vi "Verify Borders Row.vi"(7 "Column Number":i32, 8 "error in (no error)":errorcluster, 9 "No border?":bool, 10 "Column Borders IN [ ]":T1) -> (2 "Column Borders OUT [ ]":T1)   [LabVIEW 2019, in "Exaprom PDF.lvlib" / "Pdfp Table Class.lvclass"]
doc: "Version 1.0\nDeveloped by Jean-Marc Simard\nCopyright © 2010, Exaprom Inc.\nAll rights reserved.\nLicense: BSD"
uses:
  Pdfp Table Class.lvclass
  Controls/Table Controls/Border and BG Color [ ].ctl
  Controls/Table Controls/Border and BG Color.ctl
  Controls/Table Controls/Cell Border 20 px.ctl
  Exaprom PDF.lvlib
panel:
  out "error out":errorcluster
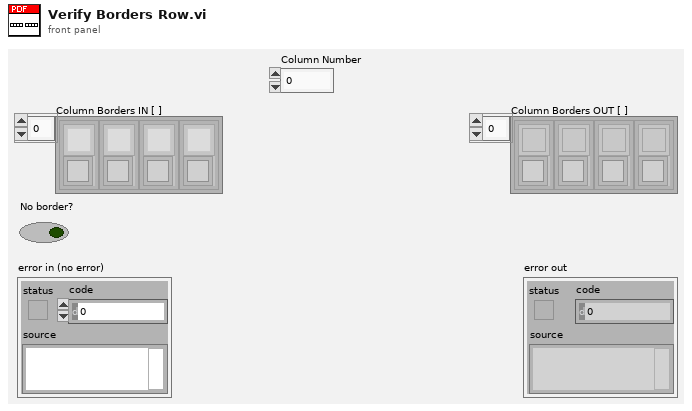
[diagram p1: front panel]
types:
  T1 = typedef "Exaprom PDF.lvlib/Border and BG Color [ ].ctl" = T2[]
  T2 = typedef "Exaprom PDF.lvlib/Border and BG Color.ctl" = cluster{"Cell Border":T3, "BG":u32}
  T3 = typedef "Exaprom PDF.lvlib/Cell Border 20 px.ctl" = u16
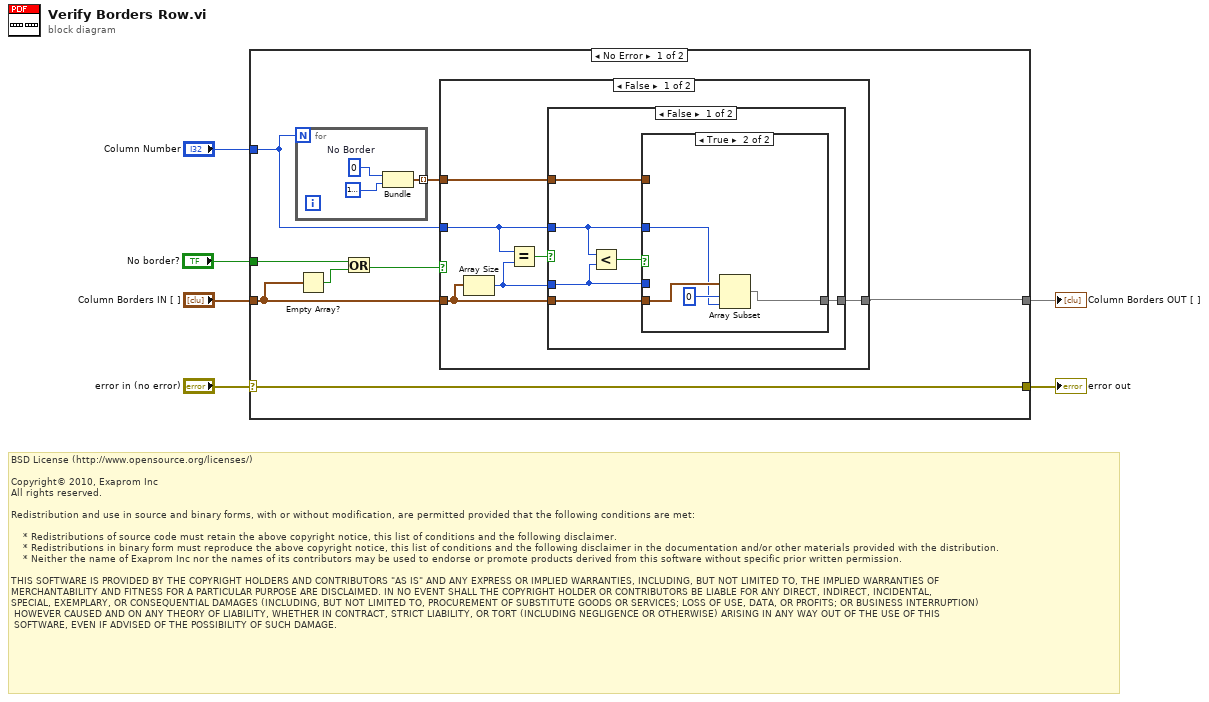
[diagram p0: block diagram]
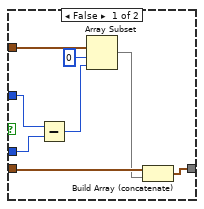
[diagram p2: hidden frame]
diagram:
  # "BSD License (http://www.opensource.org/licenses/)\n\nCopyright© 2010, Exaprom Inc\nAll rights reserved.\n\nRedistribution and use in source and binary forms, with or without modification, are permitted provided that the following conditions are met:\n\n    * Redistributions of source code must retain the above copyright notice, this list of conditions and the following disclaimer.\n    * Redistributions in binary form must reproduce the above copyright notice, this list of conditions and the following disclaimer in the documentation and/or other materials provided with the distribution.\n    * Neither the name of Exaprom Inc nor the names of its contributors may be used to endorse or promote products derived from this software without specific prior written permission.\n\nTHIS SOFTWARE IS PROVIDED BY THE COPYRIGHT HOLDERS AND CONTRIBUTORS \"AS IS\" AND ANY EXPRESS OR IMPLIED WARRANTIES, INCLUDING, BUT NOT LIMITED TO, THE IMPLIED WARRANTIES OF \nMERCHANTABILITY AND FITNESS FOR A PARTICULAR PURPOSE ARE DISCLAIMED. IN NO EVENT SHALL THE COPYRIGHT HOLDER OR CONTRIBUTORS BE LIABLE FOR ANY DIRECT, INDIRECT, INCIDENTAL,\nSPECIAL, EXEMPLARY, OR CONSEQUENTIAL DAMAGES (INCLUDING, BUT NOT LIMITED TO, PROCUREMENT OF SUBSTITUTE GOODS OR SERVICES; LOSS OF USE, DATA, OR PROFITS; OR BUSINESS INTERRUPTION)\n HOWEVER CAUSED AND ON ANY THEORY OF LIABILITY, WHETHER IN CONTRACT, STRICT LIABILITY, OR TORT (INCLUDING NEGLIGENCE OR OTHERWISE) ARISING IN ANY WAY OUT OF THE USE OF THIS\n SOFTWARE, EVEN IF ADVISED OF THE POSSIBILITY OF SUCH DAMAGE."
  n1 = case shown="No Error" "error in (no error)" {
    selector: "error in (no error)" -> [w14 w45]
    tunnel: [w14 w45] -> w5
    tunnel: "Column Borders IN [ ]" -> [w8 w44]
    tunnel: "Column Number" -> [w13 _]
    tunnel: [w12 w44] -> w3
    tunnel: "No border?" -> [w9 _]
    frame No Error {
      n2 = for {
        N: w13 -> [_]
        tunnel: [w43] -> w7 mode=indexing
        w41 = 0  # No Border
        n3 = Bundle("No Border"=w41, "Color Box"=u32 16777225) -> (w43:cluster{"No Border":i32, "Color Box":u32})  [unwired: 1 out]
      }
      n4 = Empty Array?(array=w8) -> (empty?=w11:bool)
      n5 = Or(x=w9, y=w11) -> (x .or. y?=w10:bool)
      n6 = case shown="False" w10 {
        tunnel: w8 -> [w18 _]
        tunnel: [w19 w40] -> w12
        tunnel: w7 -> [w15 w40]
        tunnel: w13 -> [w17 _]
        frame False {
          n7 = Array Size(array=w18) -> (size(s)=w16:i32)
          n8 = Equal?(x=w17, y=w16) -> (x = y?=w20:bool)
          n9 = case shown="False" w20 {
            tunnel: [w23 w39] -> w19
            tunnel: w18 -> [w25 w39]
            tunnel: w17 -> [w24 _]
            tunnel: w16 -> [w22 _]
            tunnel: w15 -> [w21 _]
            frame False {
              n10 = Less?(x=w24, y=w22) -> (x < y?=w26:bool)
              n11 = case shown="True" w26 {
                tunnel: w25 -> [w29 w38]
                tunnel: w24 -> [w34 w36]
                tunnel: [w28 w35] -> w23
                tunnel: w22 -> [w33 _]
                tunnel: w21 -> [w32 _]
                frame False {
                  n12 = Subtract(x=w34, y=w33) -> (x-y=w30:i32)
                  n13 = Array Subset(array=w32, index=0, length=w30) -> (w27:cluster{"No Border":i32, "Color Box":u32}[])
                  n14 = Build Array (concatenate)(w29, w27) -> (w28:cluster{"No Border":i32, "Color Box":u32}[])
                }
                frame True {
                  n15 = Array Subset(array=w38, index=0, length=w36) -> (w35:T1)
                }
              }
            }
            frame True {
            }
          }
        }
        frame True {
        }
      }
    }
    frame Error {
    }
  }
  "error out" <- w5
  "Column Borders OUT [ ]" <- w3
